vi "写入description.vi"(8 "error in (no error)":errorcluster caption="错误输入（无错误）", 10 "description":string="Unknown beverage", 11 "Beverage输入":refnum<class "Beverage.lvclass">) -> (0 "error out":errorcluster caption="错误输出", 3 "Beverage输出":refnum<class "Beverage.lvclass">)   [LabVIEW 2016, in "Beverage.lvclass"]
uses:
  Beverage.lvclass
  Beverage.lvclass/Beverage.ctl
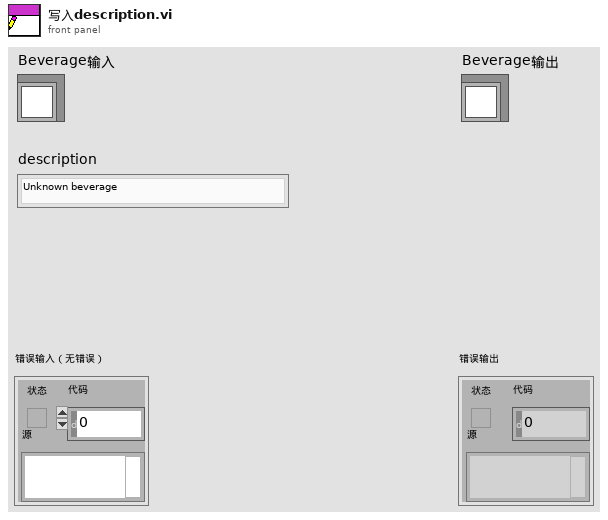
[diagram p1: front panel]
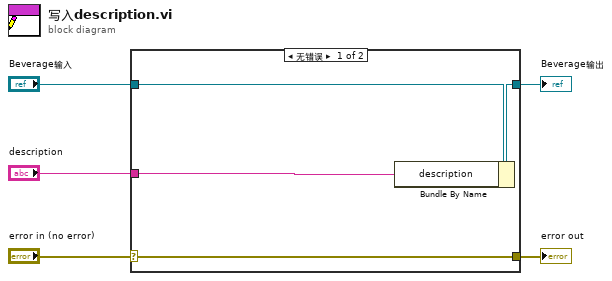
[diagram p0: block diagram]
diagram:
  n1 = case shown="无错误" "error in (no error)" {
    selector: "error in (no error)" -> [w9 w10]
    tunnel: [w9 w10] -> w4
    tunnel: [w7 w11] -> w2
    tunnel: "Beverage输入" -> [w8 w11]
    tunnel: "description" -> [w6 _]
    frame No Error {
      n2 = Bundle By Name(cluster=w8, "description"=w6) -> (w7:refnum<class "Beverage.lvclass">)
    }
    frame Error {
    }
  }
  "error out" <- w4
  "Beverage输出" <- w2
